vi "Loop Back.vi"() -> ()   [LabVIEW 2010]
panel:
  out "Boolean Array Output":bool[](array[boolean])
  in  "Boolean Array Input":bool[](array[boolean])=[FALSE, FALSE, FALSE, FALSE, FALSE]
  out "U32 Array Output":u32[](array[numeric])
  in  "U32 Array Input":u32[](array[numeric])=[0, 0, 0, 0]
  in  "Boolean Scalar Input":bool
  out "Boolean Scalar Output":bool
  out "U32 Scalar Output":u32
  in  "U32 Scalar Input":u32
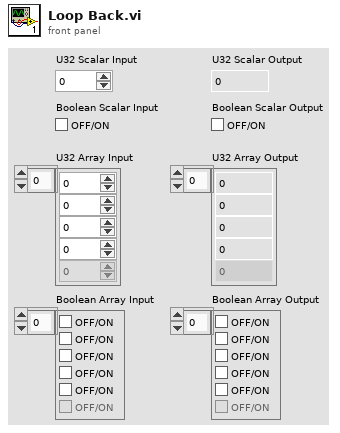
[diagram p1: front panel]
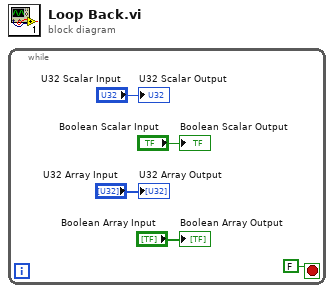
[diagram p0: block diagram]
diagram:
  n1 = while {
    stop <- FALSE stop-if-true
    "U32 Scalar Output" <- "U32 Scalar Input"
    "Boolean Scalar Output" <- "Boolean Scalar Input"
    "U32 Array Output" <- "U32 Array Input"
    "Boolean Array Output" <- "Boolean Array Input"
  }
